vi "Reinitialize.vi"(8 "error in (no error)":errorcluster, 11 "Lotis in":refnum<class "PL Lotis TII LS.lvclass">) -> (0 "error out":errorcluster, 3 "Lotis out":refnum<class "PL Lotis TII LS.lvclass">)   [LabVIEW 2015, in "PL Lotis TII LS.lvclass"]
doc: "Reinitializes connection to device based on previously specified settings."
uses:
  PL Lotis TII LS.lvclass
  PL Lotis TII LS.lvclass/PL Lotis TII LS.ctl
  <vilib>/Instr/_visa.llb/VISA Configure Serial Port (Instr).vi
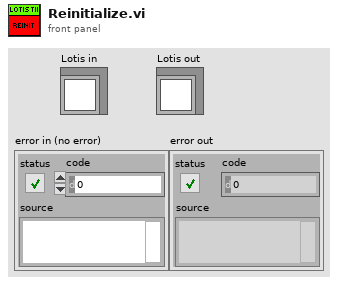
[diagram p1: front panel]
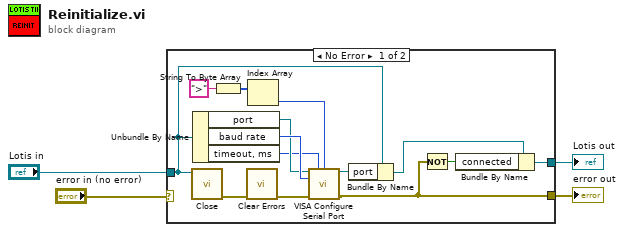
[diagram p0: block diagram]
diagram:
  n1 = case shown="No Error" "error in (no error)" {
    selector: "error in (no error)" -> [_ w19]
    tunnel: "Lotis in" -> [w18 w20]
    tunnel: [w15 w20] -> w3
    tunnel: [w7 w19] -> w2
    frame No Error {
      n2 = call "Close.vi"("Comdel in"=w18) -> ("error out"=w6:errorcluster)  [unwired: 10 in]
      n3 = Unbundle By Name(w18) -> ("port"=w13:refnum<visa-resource-name>, "baud rate"=w14:u32, "timeout, ms"=w9:u32)
      n4 = String To Byte Array(string=">") -> (unsigned byte array=w11:u8[])
      n5 = call <vilib>:"Clear Errors.vi"("error in (no error)"=w6) -> ("error out"=w5:errorcluster)  [unwired: 5 in, 1 out]
      n6 = Index Array(array=w11) -> (element=w10:u8)  [unwired: 1 in]
      n7 = call-poly "VISA Configure Serial Port"("VISA resource name"=w13, "timeout (10sec)"=w9, "termination char\n(0xA = '\\n' = LF)"=w10, "baud rate (9600)"=w14, "error in (no error)"=w5) -> ("VISA resource name out"=w8:refnum<visa-resource-name>, "error out"=w7:errorcluster)  [unwired: 9 in]
      n8 = Bundle By Name(cluster=w18, "port"=w8) -> (w17:refnum<class "PL Lotis TII LS.lvclass">)
      n9 = Not(x=w7) -> (.not. x?=w16:bool)
      n10 = Bundle By Name(cluster=w17, "connected"=w16) -> (w15:refnum<class "PL Lotis TII LS.lvclass">)
    }
    frame Error {
    }
  }
  "Lotis out" <- w3
  "error out" <- w2
